vi "Serial Daemon.vi"(8 "UUID":string, 9 "data model":refnum<class "Device Data Model.lvclass">, 10 "transmission data unit":refnum<class "Transmission Data Unit.lvclass">, 11 "serial slave":refnum<class "Serial Slave.lvclass">) -> ()   [LabVIEW 2015, in "SubVIs.lvlib" / "Serial Slave.lvclass"]
uses:
  <vilib>/Modbus/subvis/Protocol/Serial/Serial Slave/Serial Slave.lvclass
  <vilib>/Modbus/subvis/Transmission Data Unit (ADU)/Transmission Data Unit/Transmission Data Unit.lvclass
  <vilib>/Modbus/subvis/Data and Functions/Device Data Model/Device Data Model.lvclass
  <vilib>/Modbus/subvis/Protocol/Interfaces/Network Slave/Network Slave.lvclass/Network Slave.ctl
  <vilib>/Modbus/subvis/Protocol/Serial/Serial Slave/Serial Slave.lvclass/Serial Slave.ctl
  <vilib>/Modbus/subvis/Protocol/Interfaces/Network Slave/Network Slave.lvclass
panel:
  in  "stop":bool
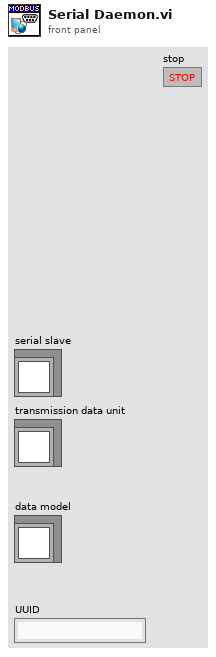
[diagram p1: front panel]
types:
  T1 = enum16{"Not Started", "Running", "Error", "Stopped"}
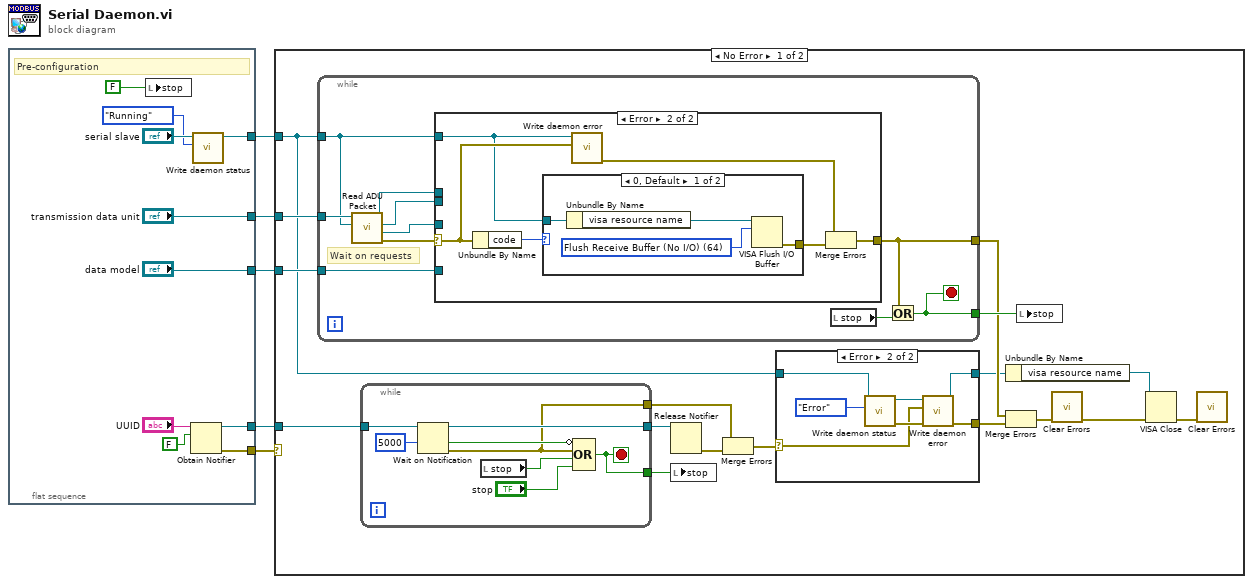
[diagram p0: block diagram]
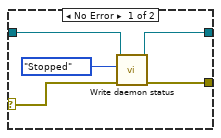
[diagram p2: hidden frame]
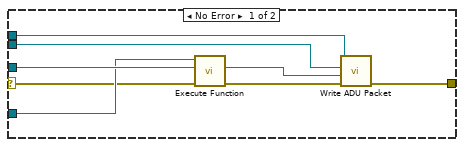
[diagram p3: hidden frame]
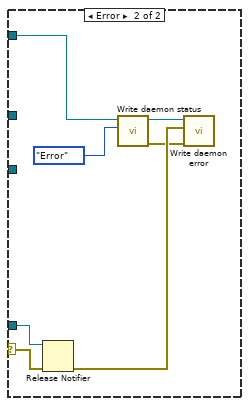
[diagram p5: hidden frame]
diagram:
  n1 = flat-sequence {
    tunnel: [w8] -> w1
    tunnel: ["transmission data unit"] -> w5
    tunnel: ["data model"] -> w4
    tunnel: [w14] -> w3
    tunnel: [w13] -> w2
    frame #0 {
      # "Pre-configuration"
      n2 = local write "stop"(FALSE ("stop")) -> ()
      n3 = Obtain Notifier(name (unnamed)="UUID", notification data type=FALSE) -> (notifier out=w13:refnum<notifier>, error out=w14:errorcluster)  [unwired: 2 in, 1 out]
      n4 = call <vilib>:"Write daemon status.vi"("daemon status"=T1."Running", "network slave in"="serial slave") -> ("network slave out"=w8:refnum<class "Serial Slave.lvclass">)  [unwired: 8 in, 1 out]
    }
  }
  n5 = case shown="No Error" w3 {
    selector: w3 -> [_ w87]
    tunnel: w5 -> [w32 _]
    tunnel: w4 -> [w31 _]
    tunnel: w1 -> [w26 w85]
    tunnel: w2 -> [w29 w86]
    frame No Error {
      n6 = while {
        tunnel: w32 -> [w62]
        tunnel: w31 -> [w60]
        tunnel: w26 -> [w54]
        tunnel: [w57] -> w30
        tunnel: [w53] -> w25
        stop <- w57 stop-if-true
        # "Wait on requests"
        n7 = call-dynamic "Read ADU Packet.vi"("protocol layer"=w54, "transmission data unit in"=w62) -> ("error out"=w61:errorcluster, "Modbus data unit"=w56:refnum<class "Modbus Data Unit (PDU).lvclass">, "protocol layer out"=w55:refnum<class "Network Protocol.lvclass">, "transmission data unit out"=w59:refnum<class "Transmission Data Unit.lvclass">)  [unwired: 5 in, 1 out]
        n8 = case shown="Error" w61 {
          selector: w61 -> [w64 w75]
          tunnel: w60 -> [w65 _]
          tunnel: w59 -> [w70 _]
          tunnel: w56 -> [w69 _]
          tunnel: w55 -> [w66 _]
          tunnel: w54 -> [_ w74]
          tunnel: [w63 w71] -> w53
          frame No Error {
            n9 = call-dynamic "Execute Function.vi"("error in (no error)"=w64, "Modbus request"=w69, "device data model in"=w65) -> ("error out"=w67:errorcluster, "Modbus response"=w68:refnum<class "Modbus Data Unit (PDU).lvclass">)  [unwired: 6 in, 1 out]
            n10 = call-dynamic "Write ADU Packet.vi"("error in (no error)"=w67, "Modbus data unit"=w68, "protocol layer"=w66, "transmission data unit in"=w70) -> ("error out"=w63:errorcluster)  [unwired: 5 in, 2 out]
          }
          frame Error {
            n11 = Unbundle By Name(w75) -> ("code"=w76:i32)
            n12 = case shown="0, Default" w76 {
              tunnel: w74 -> [w80 _]
              tunnel: [w77 _] -> w73
              frame 0, Default {
                w78 = u16 64 items=["Flush Receive Buffer"=16, "Write Transmit Buffer to Device"=32, "Flush Receive Buffer (No I/O)"=64, "Flush Transmit Buffer"=128] ("Mask")
                n13 = Unbundle By Name(w80) -> ("visa resource name"=w79:refnum<visa-resource-name>)
                n14 = VISA Flush I/O Buffer(VISA resource name=w79, mask (16)=w78) -> (error out=w77:errorcluster)  [unwired: 1 in, 1 out]
              }
              frame 56 {
              }
            }
            n15 = call <vilib>:"Write daemon error.vi"("daemon error"=w75, "network slave in"=w74) -> ("error out"=w72:errorcluster)  [unwired: 8 in, 1 out]
            n16 = Merge Errors(w72, w73) -> (w71:errorcluster)
          }
        }
        n17 = local read "stop"() -> (w58:bool)
        n18 = Or(x=w53, y=w58) -> (x .or. y?=w57:bool)
      }
      n19 = while {
        tunnel: w29 -> [w51]
        tunnel: [w50] -> w27
        tunnel: [w46] -> w28
        tunnel: [w45] -> w17
        stop <- w46 stop-if-true
        n20 = Wait on Notification(notifier=w51, timeout in ms (-1)=5000) -> (notifier out=w50:refnum<notifier>, timed out?=w49:bool, error out=w45:errorcluster)  [unwired: 2 in, 1 out]
        n21 = local read "stop"() -> (w48:bool)
        n22 = Compound Arithmetic op=OR(invert w49, w45, w48, "stop") -> (w46:bool)
      }
      n23 = Release Notifier(notifier=w27) -> (error out=w16:errorcluster)  [unwired: 2 in, 2 out]
      n24 = local write "stop"(w28) -> ()
      n25 = Merge Errors(w17, w16) -> (w18:errorcluster)
      n26 = case shown="Error" w18 {
        selector: w18 -> [w36 w40]
        tunnel: w26 -> [w35 w42]
        tunnel: [w34 w39] -> w24
        tunnel: [w33 w38] -> w22
        frame No Error {
          n27 = call <vilib>:"Write daemon status.vi"("error in (no error)"=w36, "daemon status"=T1."Stopped", "network slave in"=w35) -> ("error out"=w34:errorcluster, "network slave out"=w33:refnum<class "Serial Slave.lvclass">)  [unwired: 7 in]
        }
        frame Error {
          n28 = call <vilib>:"Write daemon status.vi"("daemon status"=T1."Error", "network slave in"=w42) -> ("error out"=w43:errorcluster, "network slave out"=w44:refnum<class "Serial Slave.lvclass">)  [unwired: 8 in]
          n29 = call <vilib>:"Write daemon error.vi"("error in (no error)"=w43, "daemon error"=w40, "network slave in"=w44) -> ("error out"=w39:errorcluster, "network slave out"=w38:refnum<class "Serial Slave.lvclass">)  [unwired: 7 in]
        }
      }
      n30 = Unbundle By Name(w22) -> ("visa resource name"=w21:refnum<visa-resource-name>)
      n31 = Merge Errors(w25, w24) -> (w23:errorcluster)
      n32 = local write "stop"(w30) -> ()
      n33 = call <vilib>:"Clear Errors.vi"("error in (no error)"=w23) -> ("error out"=w20:errorcluster)  [unwired: 5 in, 1 out]
      n34 = VISA Close(VISA resource name=w21, error in (no error)=w20) -> (error out=w19:errorcluster)
      n35 = call <vilib>:"Clear Errors.vi"("error in (no error)"=w19) -> ()  [unwired: 5 in, 2 out]
    }
    frame Error {
      n36 = Release Notifier(notifier=w86, error in (no error)=w87) -> (error out=w82:errorcluster)  [unwired: 1 in, 2 out]
      n37 = call <vilib>:"Write daemon status.vi"("daemon status"=T1."Error", "network slave in"=w85) -> ("error out"=w81:errorcluster, "network slave out"=w83:refnum<class "Serial Slave.lvclass">)  [unwired: 8 in]
      n38 = call <vilib>:"Write daemon error.vi"("error in (no error)"=w81, "daemon error"=w82, "network slave in"=w83) -> ()  [unwired: 7 in, 2 out]
    }
  }
